vi "transfer product.vi"(1 "channel":i8) -> ()   [LabVIEW 2023]
panel:
  in  "stop":bool
  out "channel":string
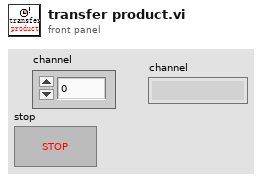
[diagram p1: front panel]
types:
  T1 = enum16{"plate1", "plate2", "plate3", "rinse", "seat"}
  T2 = enum16{"Initialize", "Absolute Position", "Relative Pickup", "Relative Dispense", "Swich valve", "Bypass"}
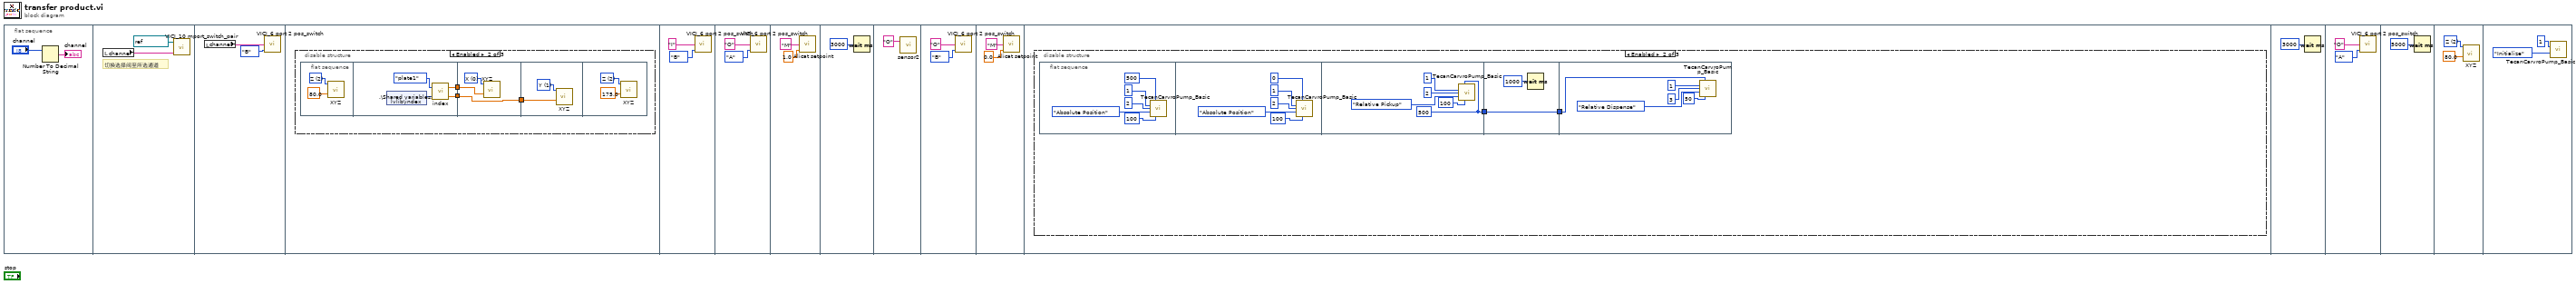
[diagram p0: block diagram]
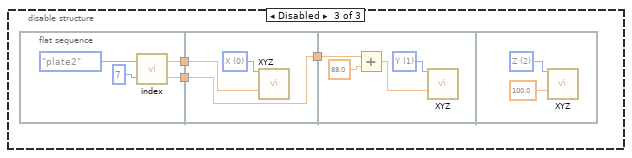
[diagram p3: hidden frame]
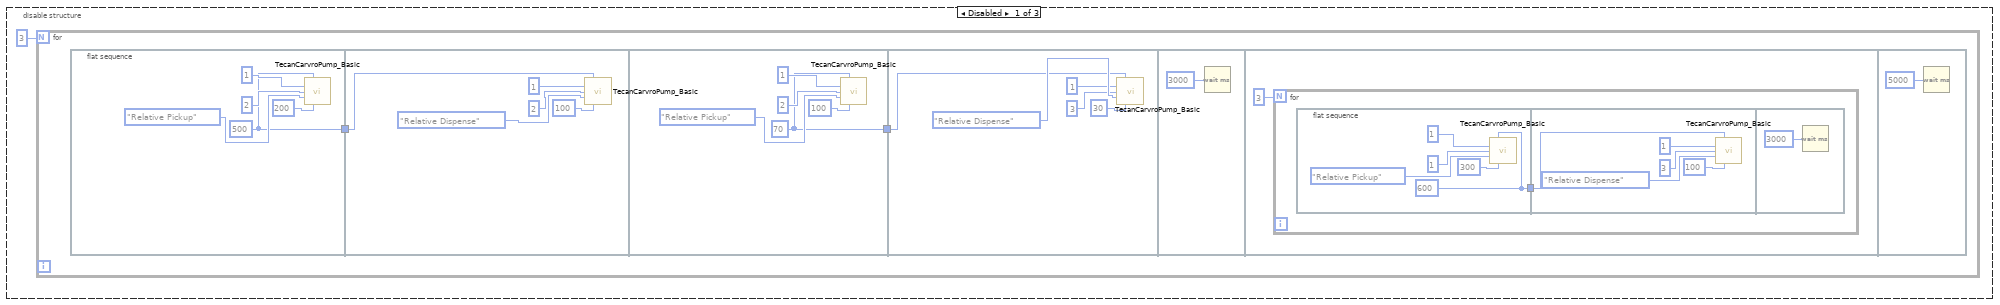
[diagram p4: hidden frame]
diagram:
  n1 = flat-sequence {
    frame #0 {
      n2 = Number To Decimal String(number="channel") -> (decimal integer string=→"channel":string)  [unwired: 1 in]
    }
    frame #1 {
      # "切换选择阀至所选通道"
      n3 = local read "channel"() -> (w4:string)
      n4 = call "VICI_10 mport_switch_pair.vi"("Go to position"=w4, "Valve COM"=refnum<visa-resource-name> "COM8") -> ()  [unwired: 2 in, 1 out]
    }
    frame #2 {
      n5 = local read "channel"() -> (w6:string)
      n6 = call "VICI_6 port 2 pos_switch.vi"("Switch to position (A/B)"=enum16{"A", "B"}."B", "Valve ID"=w6) -> ()  [unwired: 2 in, 1 out]
    }
    frame #3 {
      n7 = disable-structure shown="Enabled" {
        frame Disabled {
        }
        frame Enabled {
          n8 = flat-sequence {
            tunnel: [w14] -> w9
            tunnel: [w13] -> w8
            tunnel: w9 -> [w16]
            tunnel: w8 -> [w18]
            tunnel: [w18] -> w7
            tunnel: w7 -> [w19]
            frame #0 {
              w10 = u16 2 items=["X", "Y", "Z"] ("AXIS")
              n9 = call "XYZ.vi"("AXIS"=w10, "Set location (mm)"=80.0) -> ()  [unwired: 9 in, 5 out]
            }
            frame #1 {
              n10 = shared-variable ".\\Shared variables.lvlib\\index"() -> (w12:i8)  [unwired: 1 in, 1 out]
              n11 = call "index.vi"("index"=w12, "where"=T1."plate1") -> ("Y"=w13:dbl, "X"=w14:dbl)
            }
            frame #2 {
              w17 = u16 0 items=["X", "Y", "Z"] ("AXIS")
              n12 = call "XYZ.vi"("AXIS"=w17, "Set location (mm)"=w16) -> ()  [unwired: 9 in, 5 out]
            }
            frame #3 {
              w20 = u16 1 items=["X", "Y", "Z"] ("AXIS")
              n13 = call "XYZ.vi"("AXIS"=w20, "Set location (mm)"=w19) -> ()  [unwired: 9 in, 5 out]
            }
            frame #4 {
              w22 = u16 2 items=["X", "Y", "Z"] ("AXIS")
              n14 = call "XYZ.vi"("AXIS"=w22, "Set location (mm)"=175.0) -> ()  [unwired: 9 in, 5 out]
            }
          }
        }
        frame Disabled {
          n15 = flat-sequence {
            tunnel: [w27] -> w25
            tunnel: [w26] -> w23
            tunnel: w25 -> [w31]
            tunnel: [w30] -> w24
            tunnel: w23 -> [w30]
            tunnel: w24 -> [w33]
            frame #0 {
              n16 = call "index.vi"("index"=i8 7, "where"=T1."plate2") -> ("Y"=w26:dbl, "X"=w27:dbl)
            }
            frame #1 {
              w32 = u16 0 items=["X", "Y", "Z"] ("AXIS")
              n17 = call "XYZ.vi"("AXIS"=w32, "Set location (mm)"=w31) -> ()  [unwired: 9 in, 5 out]
            }
            frame #2 {
              w35 = u16 1 items=["X", "Y", "Z"] ("AXIS")
              n18 = Add(x=w33, y=88.0) -> (x+y=w36:dbl)
              n19 = call "XYZ.vi"("AXIS"=w35, "Set location (mm)"=w36) -> ()  [unwired: 9 in, 5 out]
            }
            frame #3 {
              w38 = u16 2 items=["X", "Y", "Z"] ("AXIS")
              n20 = call "XYZ.vi"("AXIS"=w38, "Set location (mm)"=100.0) -> ()  [unwired: 9 in, 5 out]
            }
          }
        }
      }
    }
    frame #4 {
      n21 = call "VICI_6 port 2 pos_switch.vi"("Switch to position (A/B)"=enum16{"A", "B"}."B", "Valve ID"="I") -> ()  [unwired: 2 in, 1 out]
    }
    frame #5 {
      n22 = call "VICI_6 port 2 pos_switch.vi"("Switch to position (A/B)"=enum16{"A", "B"}."A", "Valve ID"="O") -> ()  [unwired: 2 in, 1 out]
    }
    frame #6 {
      n23 = call "Alicat setpoint.vi"("Setpoint"=1.0, "Unit ID"="M") -> ()  [unwired: 3 in]
    }
    frame #7 {
      n24 = Wait (ms)(milliseconds to wait=u32 3000) -> ()  [unwired: 1 out]
    }
    frame #8 {
      n25 = call "sensor2.vi"("Sensor"="O") -> ()  [unwired: 1 in, 2 out]
    }
    frame #9 {
      n26 = call "VICI_6 port 2 pos_switch.vi"("Switch to position (A/B)"=enum16{"A", "B"}."B", "Valve ID"="O") -> ()  [unwired: 2 in, 1 out]
    }
    frame #10 {
      n27 = call "Alicat setpoint.vi"("Setpoint"=0.0, "Unit ID"="M") -> ()  [unwired: 3 in]
    }
    frame #11 {
      n28 = disable-structure shown="Enabled" {
        frame Disabled {
          n29 = for {
            N: 3 -> [_]
            n30 = flat-sequence {
              tunnel: [w54] -> w53
              tunnel: w53 -> [w59]
              tunnel: [w64] -> w52
              tunnel: w52 -> [w69]
              frame #0 {
                w54 = u16 500 ("Volume (μL)")
                n31 = call "TecanCarvroPump_Basic.vi"("Volume (μL)"=w54, "TecanPump address"=u8 1, "Valve"=u8 2, "Mode"=T2."Relative Pickup", "Speed (μL/s)"=u16 200) -> ()  [unwired: 10 in, 1 out]
              }
              frame #1 {
                n32 = call "TecanCarvroPump_Basic.vi"("Volume (μL)"=w59, "TecanPump address"=u8 1, "Valve"=u8 2, "Mode"=T2."Relative Dispense", "Speed (μL/s)"=u16 100) -> ()  [unwired: 10 in, 1 out]
              }
              frame #2 {
                w64 = u16 70 ("Volume (μL)")
                n33 = call "TecanCarvroPump_Basic.vi"("Volume (μL)"=w64, "TecanPump address"=u8 1, "Valve"=u8 2, "Mode"=T2."Relative Pickup", "Speed (μL/s)"=u16 100) -> ()  [unwired: 10 in, 1 out]
              }
              frame #3 {
                n34 = call "TecanCarvroPump_Basic.vi"("Volume (μL)"=w69, "TecanPump address"=u8 1, "Valve"=u8 3, "Mode"=T2."Relative Dispense", "Speed (μL/s)"=u16 30) -> ()  [unwired: 10 in, 1 out]
              }
              frame #4 {
                n35 = Wait (ms)(milliseconds to wait=u32 3000) -> ()  [unwired: 1 out]
              }
              frame #5 {
                n36 = for {
                  N: 3 -> [_]
                  n37 = flat-sequence {
                    tunnel: [w77] -> w76
                    tunnel: w76 -> [w82]
                    frame #0 {
                      w77 = u16 600 ("Volume (μL)")
                      n38 = call "TecanCarvroPump_Basic.vi"("Volume (μL)"=w77, "TecanPump address"=u8 1, "Valve"=u8 1, "Mode"=T2."Relative Pickup", "Speed (μL/s)"=u16 300) -> ()  [unwired: 10 in, 1 out]
                    }
                    frame #1 {
                      n39 = call "TecanCarvroPump_Basic.vi"("Volume (μL)"=w82, "TecanPump address"=u8 1, "Valve"=u8 3, "Mode"=T2."Relative Dispense", "Speed (μL/s)"=u16 100) -> ()  [unwired: 10 in, 1 out]
                    }
                    frame #2 {
                      n40 = Wait (ms)(milliseconds to wait=u32 3000) -> ()  [unwired: 1 out]
                    }
                  }
                }
              }
              frame #6 {
                n41 = Wait (ms)(milliseconds to wait=u32 5000) -> ()  [unwired: 1 out]
              }
            }
          }
        }
        frame Enabled {
          n42 = flat-sequence {
            tunnel: [w101] -> w90
            tunnel: w90 -> [w107]
            tunnel: [w107] -> w89
            tunnel: w89 -> [w108]
            frame #0 {
              n43 = call "TecanCarvroPump_Basic.vi"("Volume (μL)"=u16 500, "TecanPump address"=u8 1, "Valve"=u8 2, "Mode"=T2."Absolute Position", "Speed (μL/s)"=u16 100) -> ()  [unwired: 10 in, 1 out]
            }
            frame #1 {
              n44 = call "TecanCarvroPump_Basic.vi"("Volume (μL)"=u16 0, "TecanPump address"=u8 1, "Valve"=u8 2, "Mode"=T2."Absolute Position", "Speed (μL/s)"=u16 100) -> ()  [unwired: 10 in, 1 out]
            }
            frame #2 {
              w101 = u16 500 ("Volume (μL)")
              n45 = call "TecanCarvroPump_Basic.vi"("Volume (μL)"=w101, "TecanPump address"=u8 1, "Valve"=u8 2, "Mode"=T2."Relative Pickup", "Speed (μL/s)"=u16 100) -> ()  [unwired: 10 in, 1 out]
            }
            frame #3 {
              n46 = Wait (ms)(milliseconds to wait=u32 1000) -> ()  [unwired: 1 out]
            }
            frame #4 {
              n47 = call "TecanCarvroPump_Basic.vi"("Volume (μL)"=w108, "TecanPump address"=u8 1, "Valve"=u8 3, "Mode"=T2."Relative Dispense", "Speed (μL/s)"=u16 50) -> ()  [unwired: 10 in, 1 out]
            }
          }
        }
        frame Disabled {
        }
      }
    }
    frame #12 {
      n48 = Wait (ms)(milliseconds to wait=u32 3000) -> ()  [unwired: 1 out]
    }
    frame #13 {
      n49 = call "VICI_6 port 2 pos_switch.vi"("Switch to position (A/B)"=enum16{"A", "B"}."A", "Valve ID"="O") -> ()  [unwired: 2 in, 1 out]
    }
    frame #14 {
      n50 = Wait (ms)(milliseconds to wait=u32 5000) -> ()  [unwired: 1 out]
    }
    frame #15 {
      w118 = u16 2 items=["X", "Y", "Z"] ("AXIS")
      n51 = call "XYZ.vi"("AXIS"=w118, "Set location (mm)"=80.0) -> ()  [unwired: 9 in, 5 out]
    }
    frame #16 {
      n52 = call "TecanCarvroPump_Basic.vi"("TecanPump address"=u8 1, "Mode"=T2."Initialize") -> ()  [unwired: 13 in, 1 out]
    }
  }
